vi "FactoryCreate.vi"(0 "reference in":refnum<class "UseCaseDiagramGraph.lvclass">, 5 "error in (no error)":errorcluster) -> (14 "reference out":refnum<class "UseCaseDiagramGraph.lvclass">, 19 "error out":errorcluster)   [LabVIEW 2016, in "UseCaseDiagramGraph.lvclass"]
uses:
  <resource>/Framework/Providers/Open_GDS/UML/UseCaseDiagramGraph_class/UseCaseDiagramGraph.lvclass
  <resource>/Framework/Providers/Open_GDS/UML/UseCaseDiagramGraph_class/UseCaseDiagramGraph.lvclass/UseCaseDiagramGraph.ctl
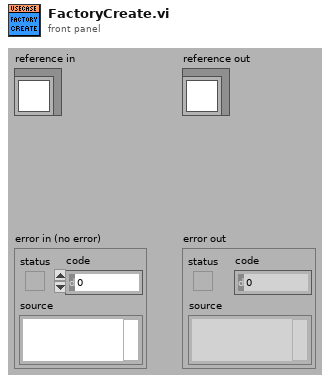
[diagram p1: front panel]
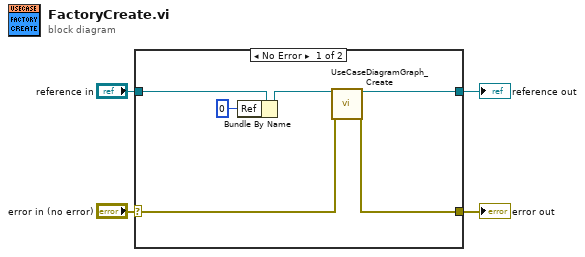
[diagram p0: block diagram]
diagram:
  n1 = case shown="No Error" "error in (no error)" {
    selector: "error in (no error)" -> [w6 w12]
    tunnel: [w5 w12] -> w3
    tunnel: [w10 w11] -> w1
    tunnel: "reference in" -> [w9 w11]
    frame No Error {
      n2 = Bundle By Name(cluster=w9, "Ref"=u32 0) -> (w8:refnum<class "UseCaseDiagramGraph.lvclass">)
      n3 = call <resource>:"UseCaseDiagramGraph_Create.vi"("reference"=w8, "error in (no error)"=w6) -> ("reference out"=w10:refnum<class "UseCaseDiagramGraph.lvclass">, "error out"=w5:errorcluster)  [unwired: 16 in]
    }
    frame Error {
    }
  }
  "error out" <- w3
  "reference out" <- w1
